vi "Excel Write Header.vi"(8 "error in":errorcluster, 10 "Header Data":string[][](array[string]), 11 "_Worksheet In":refnum<k7>) -> (0 "error out":errorcluster, 2 "Header Size":i32, 3 "_Worksheet Out":refnum<k7>)   [LabVIEW 2012]
doc: "Formats the data file header of an Excel Worksheet.\n\nHeader should be 2D array with equal lengths in Comments array and Channel Names array.\nComments array will be merged to one cell.\n\nReturns number of rows used by header."
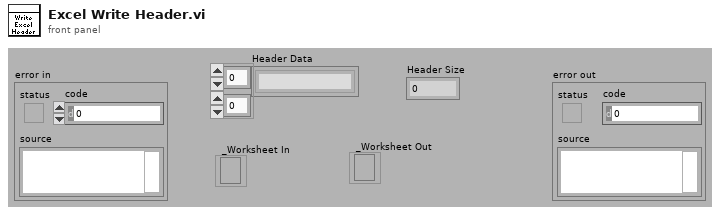
[diagram p1: front panel]
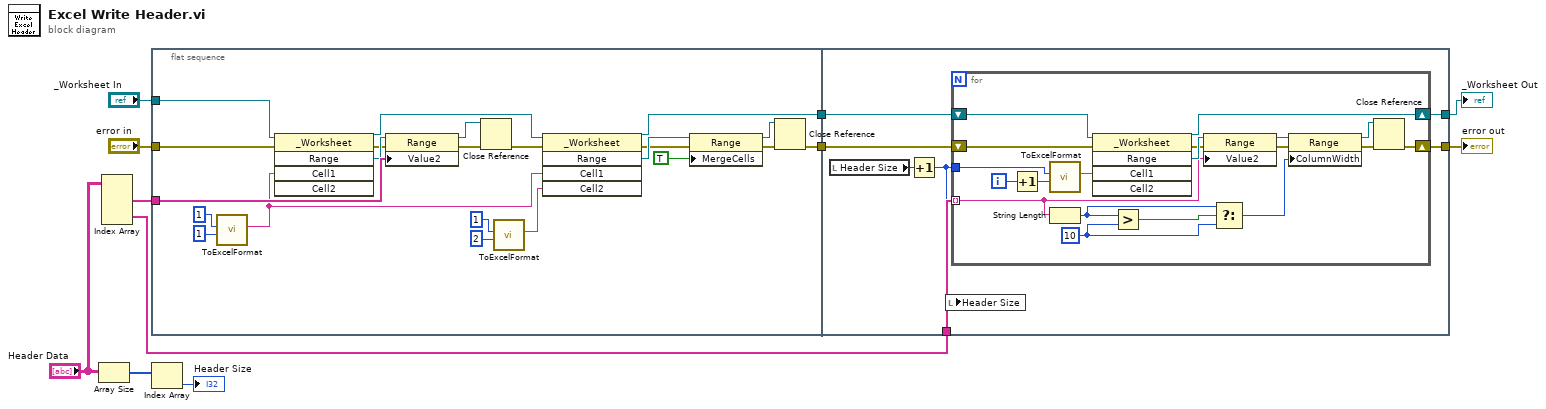
[diagram p0: block diagram]
diagram:
  n1 = Array Size(array="Header Data") -> (size(s)=w2:i32[])
  n2 = Index Array(array="Header Data") -> (element #1=w7:string[], element #2=w6:string[])  [unwired: 4 in]
  n3 = flat-sequence {
    tunnel: "_Worksheet In" -> [w33]
    tunnel: "error in" -> [w32]
    tunnel: w7 -> [w31]
    tunnel: [w14] -> w9
    tunnel: [w15] -> w8
    tunnel: w9 -> [w40]
    tunnel: w8 -> [w39]
    tunnel: w6 -> [w38]
    tunnel: [w37] -> w5
    tunnel: [w36] -> w4
    frame #0 {
      n4 = call "ToExcelFormat.vi"("Column"=1, "Row"=1) -> ("Output String"=w13:string)  [unwired: 9 in]
      n5 = invoke class="_Worksheet" method="Range"(reference=w33, error in=w32, "Cell1"=w13) -> (reference out=w19:refnum<k7>, error out=w28:errorcluster, "Range"=w30:refnum<k7>)  [unwired: 2 in, 2 out]
      n6 = property class="Range"(reference=w30, error in=w28, "Value2"=w31) -> (reference out=w29:refnum<k7>, error out=w27:errorcluster)
      n7 = Close Reference(reference=w29, error in (no error)=w27) -> (error out=w18:errorcluster)
      n8 = call "ToExcelFormat.vi"("Column"=2, "Row"=1) -> ("Output String"=w12:string)  [unwired: 9 in]
      n9 = invoke class="_Worksheet" method="Range"(reference=w19, error in=w18, "Cell1"=w13, "Cell2"=w12) -> (reference out=w14:refnum<k7>, error out=w23:errorcluster, "Range"=w24:refnum<k7>)  [unwired: 1 in, 2 out]
      n10 = property class="Range"(reference=w24, error in=w23, "MergeCells"=TRUE) -> (reference out=w17:refnum<k7>, error out=w16:errorcluster)
      n11 = Close Reference(reference=w17, error in (no error)=w16) -> (error out=w15:errorcluster)
    }
    frame #1 {
      n12 = local read "Header Size"() -> (w35:i32)
      n13 = Increment(x=w35) -> (x+1=w34:i32)
      n14 = local write "Header Size"(w34) -> ()
      n15 = for {
        shift-right: [w55] -> w37
        shift-left: w39 -> [w57]
        shift-right: [w54] -> w36
        shift-left: w40 -> [w59]
        tunnel: w38 -> [w45] mode=indexing
        tunnel: w34 -> [w50]
        i -> [w52]
        w43 = 10 ("y")
        n16 = Increment(x=w52) -> (x+1=w51:i32)
        n17 = call "ToExcelFormat.vi"("Column"=w51, "Row"=w50) -> ("Output String"=w53:string)  [unwired: 9 in]
        n18 = String Length(string=w45) -> (length=w42:i32)
        n19 = invoke class="_Worksheet" method="Range"(reference=w59, error in=w57, "Cell1"=w53) -> (reference out=w54:refnum<k7>, error out=w56:errorcluster, "Range"=w58:refnum<k7>)  [unwired: 2 in, 2 out]
        n20 = Greater?(x=w42, y=w43) -> (0:w44:bool)
        n21 = property class="Range"(reference=w58, error in=w56, "Value2"=w45) -> (reference out=w49:refnum<k7>, error out=w48:errorcluster)
        n22 = Select(t=w42, s=w44, f=w43) -> (s? t:f=w41:i32)
        n23 = property class="Range"(reference=w49, error in=w48, "ColumnWidth"=w41) -> (reference out=w47:refnum<k7>, error out=w46:errorcluster)
        n24 = Close Reference(reference=w47, error in (no error)=w46) -> (error out=w55:errorcluster)
      }
    }
  }
  n25 = Index Array(array=w2) -> (element=→"Header Size":i32)  [unwired: 1 in]
  "_Worksheet Out" <- w4
  "error out" <- w5
